vi "PUT.vi"   [LabVIEW 2020, in "Library Commun.lvlib" / "Library Http.lvlib" / "Session.lvclass"]
doc: "Creates or updates data and sends it to the URL you specify.\n\nUnlike a POST request, PUT requests require all available property and attribute values to be present because the PUT request updates all data within the resource. Adding all available property and attribute values will guarantee that the operation can be performed multiple times without changing the result beyond the initial application."
uses:
  Session.lvclass
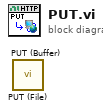
[diagram p0: block diagram]
diagram:
  n1 = call "PUT (File).vi"() -> ()  [unwired: 7 in, 5 out]
  n2 = call "PUT (Buffer).vi"() -> ()  [unwired: 7 in, 5 out]
